vi "Derivative (single).vi"(8 "error in (no error)":errorcluster, 9 "Type":enum16{"dy/dx vs x", "dx/dy vs y"}(ring), 11 "XY-data":cluster{"X-array":dbl[], "Y-array":dbl[]}) -> (0 "error out":errorcluster, 2 "Differential out":cluster{"X-array":dbl[], "Y-array":dbl[]} {"Y-array" format="%.2p"; "X-array" format="%.2p"}, 3 "XY-data out":cluster{"X-array":dbl[], "Y-array":dbl[]})   [LabVIEW 2016, in "xy_utilities.lvlib"]
doc: "Performs numerical differentiation of <b>XY-data</b> using the finite difference method.\n\n<b>Interval</b> is the range over which the finite difference is calculated.\n<b>Interval Units</b> defines the units of the <b>Interval</b> to be the number of points or the same units as the x (or y) data.\n<b>Type</b> specifies taking a derivative with respect to x or y.\n\nWire data to the data input to determine the polymorphic instance to use or manually select the instance."
uses:
  xy_utilities.lvlib
  Swap X and Y (single).vi
  <vilib>/Analysis/NI_AALPro.lvlib
panel:
  in  "Interval Units":enum16{"Points", "Data"}(ring)
  in  "Interval (h)":dbl=2.0
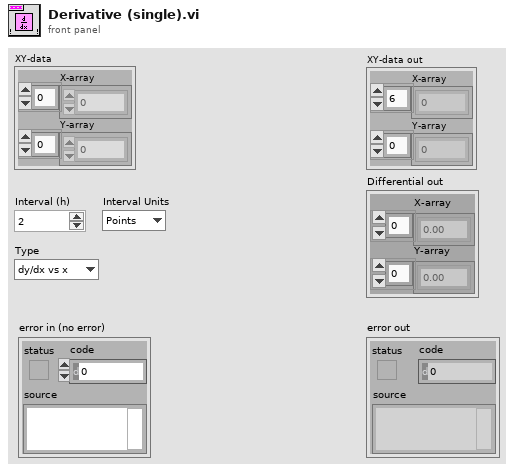
[diagram p1: front panel]
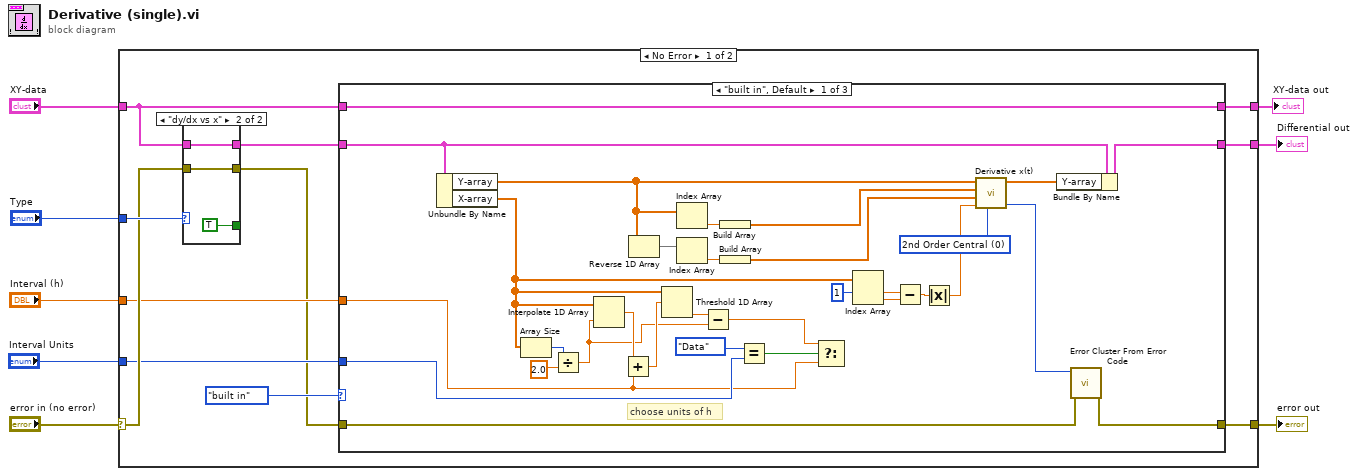
[diagram p0: block diagram]
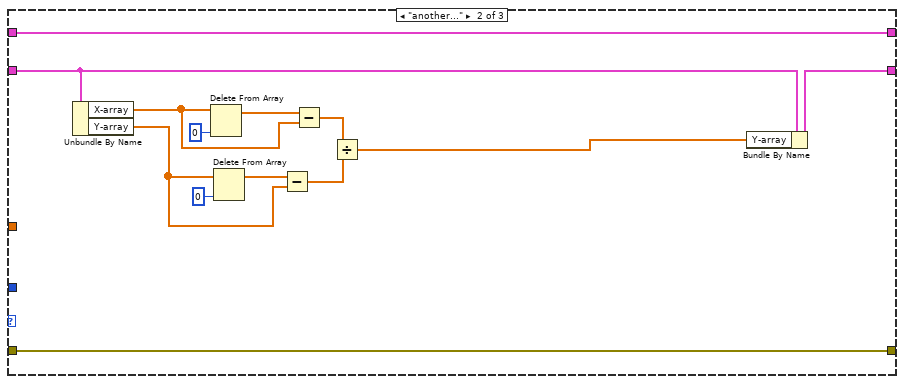
[diagram p2: hidden frame]
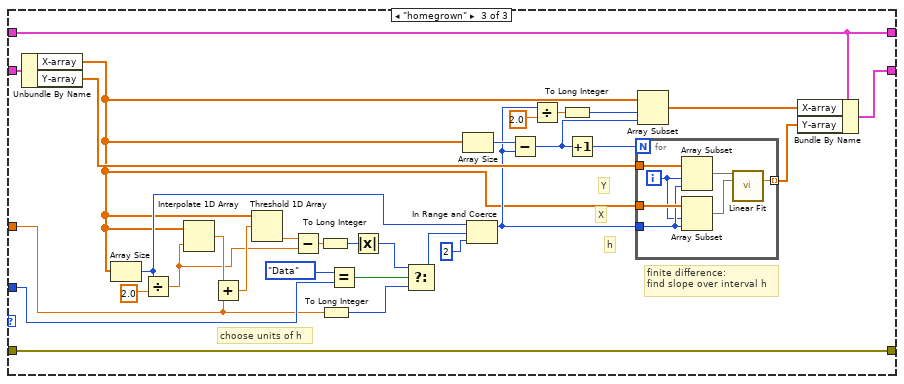
[diagram p3: hidden frame]
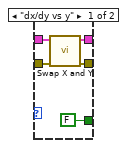
[diagram p4: hidden frame]
diagram:
  n1 = case shown="No Error" "error in (no error)" {
    selector: "error in (no error)" -> [w18 w111]
    tunnel: [w11 w111] -> w7
    tunnel: "XY-data" -> [w17 w110]
    tunnel: [w16 _] -> w5
    tunnel: "Type" -> [w19 _]
    tunnel: "Interval (h)" -> [w14 _]
    tunnel: [w12 w110] -> w2
    tunnel: "Interval Units" -> [w13 _]
    frame No Error {
      n2 = case shown="\"dy/dx vs x\"" w19 {
        tunnel: w17 -> [w106 w109]
        tunnel: [w105 w109] -> w15
        tunnel: [w104 w108] -> w9
        tunnel: w18 -> [w103 w108]
        tunnel: [FALSE ("dy/dx vs x") TRUE ("dy/dx vs x")] -> _
        frame "dx/dy vs y" {
          n3 = call-poly "Swap X and Y.vi"("error in (no error)"=w103, "XY-data"=w106) -> ("error out"=w104:errorcluster, "XY-data out"=w105:cluster{"X-array":dbl[], "Y-array":dbl[]})  [unwired: 8 in]
        }
        frame "dy/dx vs x" {
        }
      }
      n4 = case shown="\"built in\", Default" enum16{"built in", "another...", "homegrown"}."built in" ("Subset Method") {
        tunnel: w17 -> [w46 w62 w76]
        tunnel: [w37 w54 w82] -> w16
        tunnel: w15 -> [w47 w56 w64]
        tunnel: w14 -> [w27 _ w65]
        tunnel: w13 -> [w28 _ w66]
        tunnel: [w46 w62 w76] -> w12
        tunnel: [w48 w63 w75] -> w11
        tunnel: w9 -> [w49 w63 w75]
        frame "built in", Default {
          w44 = u16 0 items=["2nd Order Central", "4th Order Central", "Forward", "Backward"] ("method")
          # "choose units of h"
          n5 = Unbundle By Name(w47) -> ("Y-array"=w43:dbl[], "X-array"=w25:dbl[])
          n6 = Array Size(array=w25) -> (size(s)=w31:i32)
          n7 = Divide(x=w31, y=2.0) -> (x/y=w29:dbl)
          n8 = Interpolate 1D Array(1:w29, 2:w25) -> (0:w30:dbl)
          n9 = Add(x=w30, y=w27) -> (x+y=w34:dbl)
          n10 = Reverse 1D Array(array=w43) -> (reversed array=w42:dbl[])
          n11 = Threshold 1D Array(2:w34, 3:w25) -> (0:w35:dbl)  [unwired: 1 in]
          n12 = Index Array(array=w43) -> (element=w40:dbl)  [unwired: 1 in]
          n13 = Index Array(array=w42) -> (element=w41:dbl)  [unwired: 1 in]
          n14 = Subtract(x=w35, y=w29) -> (x-y=w26:dbl)
          n15 = Build Array(w40) -> (w39:dbl[])
          n16 = Build Array(w41) -> (w38:dbl[])
          n17 = Equal?(x=enum16{"Points", "Data"}."Data" ("Interval Units"), y=w28) -> (x = y?=w32:bool)
          n18 = Select(t=w26, s=w32, f=w27) -> ()  [unwired: 1 out]
          n19 = Index Array(array=w25, index #1=1 ("index")) -> (element #1=w23:dbl, element #2=w24:dbl)  [unwired: 1 in]
          n20 = Subtract(x=w23, y=w24) -> (x-y=w22:dbl)
          n21 = Absolute Value(x=w22) -> (abs(x)=w20:dbl)
          n22 = call <vilib>:"Derivative x(t).vi"("method"=w44, "dt"=w20, "Final Condition"=w38, "Initial Condition"=w39, "X"=w43) -> ("error"=w50:i32, "dX/dt"=w45:dbl[])  [unwired: 5 in]
          n23 = Bundle By Name(cluster=w47, "Y-array"=w45) -> (w37:cluster{"X-array":dbl[], "Y-array":dbl[]})
          n24 = call <vilib>:"Error Cluster From Error Code.vi"("error in (no error)"=w49, "error code (0)"=w50) -> ("error out"=w48:errorcluster)  [unwired: 7 in]
        }
        frame "another..." {
          n25 = Unbundle By Name(w56) -> ("X-array"=w51:dbl[], "Y-array"=w59:dbl[])
          n26 = Delete From Array(array=w51, index=0) -> (array with subset deleted=w61:dbl[])  [unwired: 1 in, 1 out]
          n27 = Delete From Array(array=w59, index=0) -> (array with subset deleted=w60:dbl[])  [unwired: 1 in, 1 out]
          n28 = Subtract(x=w60, y=w59) -> (x-y=w57:dbl[])
          n29 = Subtract(x=w61, y=w51) -> (x-y=w58:dbl[])
          n30 = Divide(x=w58, y=w57) -> (x/y=w55:dbl[])
          n31 = Bundle By Name(cluster=w56, "Y-array"=w55) -> (w54:cluster{"X-array":dbl[], "Y-array":dbl[]})
        }
        frame "homegrown" {
          # "choose units of h"
          # "h"
          # "finite difference:\nfind slope over interval h"
          # "Y"
          # "X"
          n32 = Unbundle By Name(w64) -> ("X-array"=w67:dbl[], "Y-array"=w77:dbl[])
          n33 = Array Size(array=w67) -> (size(s)=w74:i32)
          n34 = Divide(x=w74, y=2.0) -> (x/y=w68:dbl)
          n35 = Interpolate 1D Array(1:w68, 2:w67) -> (0:w69:dbl)
          n36 = Add(x=w69, y=w65) -> (x+y=w84:dbl)
          n37 = Threshold 1D Array(2:w84, 3:w67) -> (0:w86:dbl)  [unwired: 1 in]
          n38 = Subtract(x=w86, y=w68) -> (x-y=w85:dbl)
          n39 = To Long Integer(number=w85) -> (32bit integer=w83:i32)
          n40 = To Long Integer(number=w65) -> (32bit integer=w79:i32)
          n41 = Equal?(x=enum16{"Points", "Data"}."Data" ("Interval Units"), y=w66) -> (x = y?=w80:bool)
          n42 = Absolute Value(x=w83) -> (abs(x)=w72:i32)
          n43 = Select(t=w72, s=w80, f=w79) -> (s? t:f=w71:i32)
          n44 = Array Size(array=w67) -> (size(s)=w90:i32)
          n45 = In Range and Coerce(upper limit=w74, x=w71, lower limit=2) -> (coerced(x)=w70:i32)  [unwired: 1 out]
          n46 = Subtract(x=w90, y=w70) -> (x-y=w93:i32)
          n47 = Divide(x=w70, y=2.0) -> (x/y=w88:dbl)
          n48 = To Long Integer(number=w88) -> (32bit integer=w94:i32)
          n49 = Increment(x=w93) -> (x+1=w91:i32)
          n50 = for {
            N: w91 -> [_]
            tunnel: w77 -> [w101]
            tunnel: w67 -> [w100]
            tunnel: w70 -> [w99]
            tunnel: [w98] -> w78 mode=indexing
            i -> [w95]
            n51 = Array Subset "Array Subset"(array=w101, index=w95, length=w99) -> (w97:dbl[])
            n52 = Array Subset(array=w100, index=w95, length=w99) -> (w96:dbl[])
            n53 = call <vilib>:"Linear Fit.vi"("Y"=w97, "X"=w96) -> ("slope"=w98:dbl)  [unwired: 9 in, 4 out]
          }
          n54 = Array Subset(array=w67, index=w94, length=w93) -> (w92:dbl[])
          n55 = Bundle By Name(cluster=w76, "X-array"=w92, "Y-array"=w78) -> (w82:cluster{"X-array":dbl[], "Y-array":dbl[]})
        }
      }
    }
    frame Error {
    }
  }
  "error out" <- w7
  "Differential out" <- w5
  "XY-data out" <- w2
